vi "BasicExampleMux.vi"() -> ()   [LabVIEW 2025]
uses:
  PalmSens/PalmSens.lvclass
  C:/Users/stef/code/palmsenssdk/labview/PalmSens/Libraries/PalmSens.Core.Simplified.LabVIEW.dll
  PalmSens/Libraries/PalmSens.Core.Simplified.LabVIEW.dll
  PalmSens/MeasurementResults.ctl
  PalmSens/LiveCurveResult.ctl
panel:
  out "NumMuxChannels":i32
  out "Results":T1
  out "LSV Method Indicator":refnum<k24>
  out "Array":string[](array[string])
  out "Is Measuring":bool
  in  "PalmSens.lvclass":refnum<class "PalmSens.lvclass">
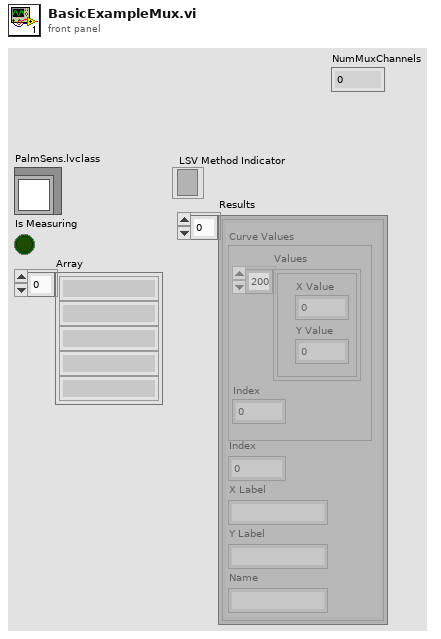
[diagram p1: front panel]
types:
  T1 = typedef "MeasurementResults.ctl" = T2[]
  T2 = typedef "LiveCurveResult.ctl" = cluster{"X Label":string, "Y Label":string, "Name":string, "Index":i16, "Curve Values":cluster{"Values":cluster{"X Value":dbl, "Y Value":dbl}[], "Index":i16}}
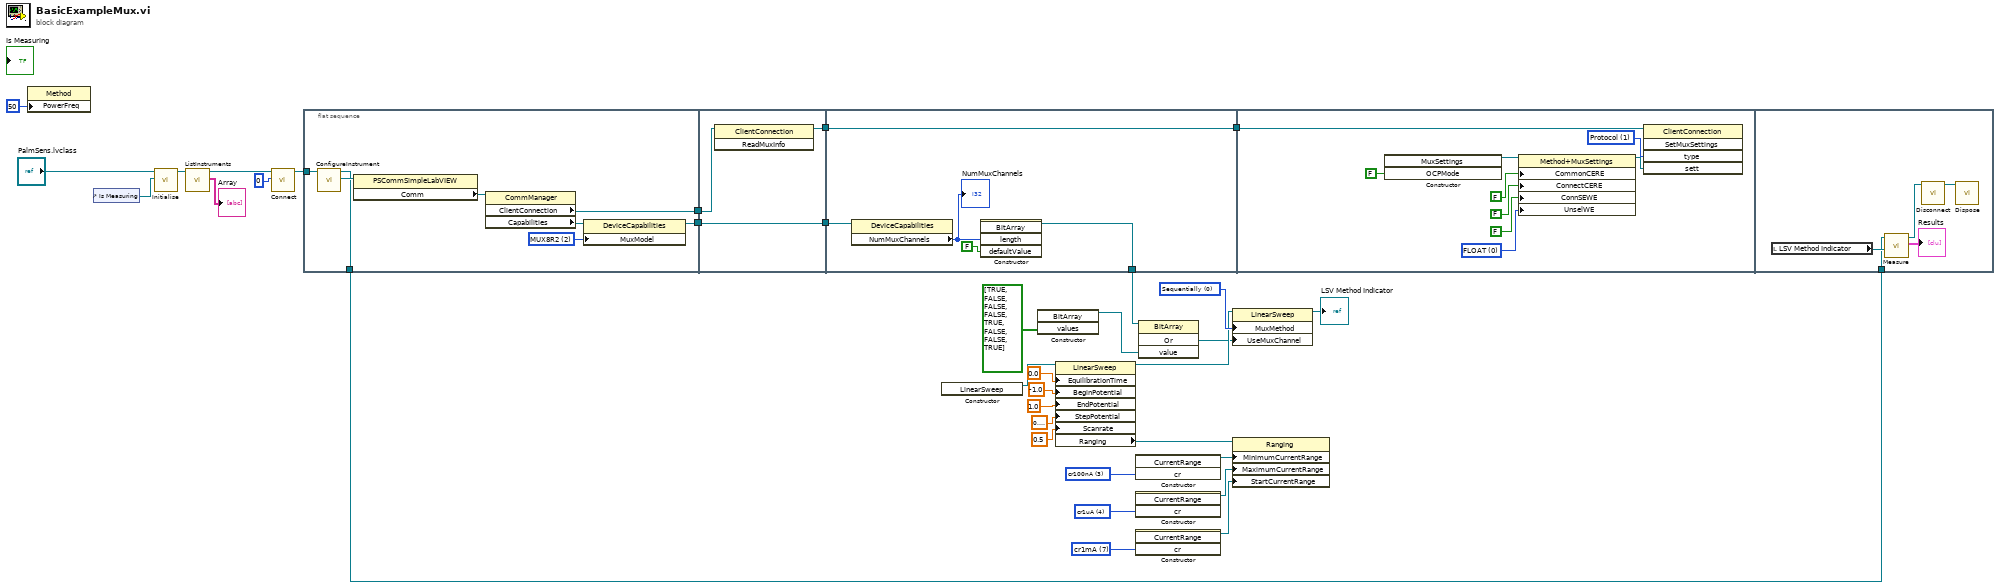
[diagram p0: block diagram]
diagram:
  w22 = 0 items=["Sequentially"=0, "Alternatingly"=1, "None"=-1] ("MuxMethod")
  w25 = 4 items=["cr100pA"=0, "cr1nA"=1, "cr10nA"=2, "cr100nA"=3, "cr1uA"=4, "cr10uA"=5, "cr100uA"=6, "cr1mA"=7, "cr10mA"=8, "cr100mA"=9, "cr2uA"=10, "cr4uA"=11, "cr8uA"=12, "cr16uA"=13, "cr32uA"=14, "cr125uA"=17, "cr250uA"=18, "cr500uA"=19, "cr5mA"=20, "cr6uA"=21, "cr13uA"=22, "cr25uA"=23, "cr50uA"=24, "cr200uA"=25, "cr63uA"=26] ("cr")
  w26 = 7 items=["cr100pA"=0, "cr1nA"=1, "cr10nA"=2, "cr100nA"=3, "cr1uA"=4, "cr10uA"=5, "cr100uA"=6, "cr1mA"=7, "cr10mA"=8, "cr100mA"=9, "cr2uA"=10, "cr4uA"=11, "cr8uA"=12, "cr16uA"=13, "cr32uA"=14, "cr125uA"=17, "cr250uA"=18, "cr500uA"=19, "cr5mA"=20, "cr6uA"=21, "cr13uA"=22, "cr25uA"=23, "cr50uA"=24, "cr200uA"=25, "cr63uA"=26] ("cr")
  w28 = 3 items=["cr100pA"=0, "cr1nA"=1, "cr10nA"=2, "cr100nA"=3, "cr1uA"=4, "cr10uA"=5, "cr100uA"=6, "cr1mA"=7, "cr10mA"=8, "cr100mA"=9, "cr2uA"=10, "cr4uA"=11, "cr8uA"=12, "cr16uA"=13, "cr32uA"=14, "cr125uA"=17, "cr250uA"=18, "cr500uA"=19, "cr5mA"=20, "cr6uA"=21, "cr13uA"=22, "cr25uA"=23, "cr50uA"=24, "cr200uA"=25, "cr63uA"=26] ("cr")
  n1 = property class="Method"("PowerFreq"=50) -> ()  [unwired: 2 in, 2 out]
  n2 = control-ref of="Is Measuring"() -> (w33:refnum<vi>)
  n3 = call-dynamic "Initialise.vi"("Is Measuring Refnum"=w33, "PalmSens in"="PalmSens.lvclass") -> ("PalmSens out"=w32:refnum<class "PalmSens.lvclass">)  [unwired: 8 in, 1 out]
  n4 = call-dynamic "ListInstruments.vi"("PalmSens in"=w32) -> ("Array"=→"Array":string[], "PalmSens out"=w30:refnum<class "PalmSens.lvclass">)  [unwired: 8 in, 1 out]
  n5 = call-dynamic "Connect.vi"("Instrument Index"=0, "PalmSens in"=w30) -> ("PalmSens out"=w2:refnum<class "PalmSens.lvclass">)  [unwired: 8 in, 1 out]
  n6 = flat-sequence {
    tunnel: [w39] -> w11
    tunnel: [w38] -> w8
    tunnel: w2 -> [w37]
    tunnel: [w35] -> w1
    tunnel: [w44] -> w10
    tunnel: w11 -> [w45]
    tunnel: w8 -> [w43]
    tunnel: [w43] -> w7
    tunnel: w10 -> [w50]
    tunnel: [w50] -> w9
    tunnel: w7 -> [w49]
    tunnel: [w46] -> w5
    tunnel: w9 -> [w51]
    tunnel: w1 -> [w60]
    frame #0 {
      w40 = 2 items=["MUX8", "MUX16", "MUX8R2", "PicoMUX16", "PicoMUX256"] ("MuxModel")
      n7 = call-dynamic "ConfigureInstrument.vi"("PalmSens in"=w37) -> ("PSLabView Instance"=w36:refnum<k24>, "PalmSens out"=w35:refnum<class "PalmSens.lvclass">)  [unwired: 8 in, 1 out]
      n8 = property class="PSCommSimpleLabVIEW"(reference=w36) -> ("Comm"=w41:refnum<k24>)  [unwired: 1 in, 2 out]
      n9 = property class="CommManager"(reference=w41) -> ("ClientConnection"=w39:refnum<k24>, "Capabilities"=w42:refnum<k24>)  [unwired: 1 in, 2 out]
      n10 = property class="DeviceCapabilities"(reference=w42, "MuxModel"=w40) -> (reference out=w38:refnum<k24>)  [unwired: 1 in, 1 out]
    }
    frame #1 {
      n11 = invoke class="ClientConnection" method="ReadMuxInfo"(reference=w45) -> (reference out=w44:refnum<k24>)  [unwired: 2 in, 2 out]
    }
    frame #2 {
      n12 = property class="DeviceCapabilities"(reference=w49) -> ("NumMuxChannels"=w48:i32)  [unwired: 1 in, 2 out]
      "NumMuxChannels" <- w48
      n13 = constructor class="BitArray"("length"=w48, "defaultValue"=FALSE) -> (reference out=w46:refnum<k24>)  [unwired: 3 in, 4 out]
    }
    frame #3 {
      w54 = 0 items=["FLOAT", "GND", "VSTDBY"] ("UnselWE")
      w52 = 1 items=["AuxAddress", "Protocol"] ("type")
      n14 = constructor class="Method+MuxSettings"("OCPMode"=FALSE) -> (reference out=w58:refnum<k24>)  [unwired: 3 in, 3 out]
      n15 = property class="Method+MuxSettings"(reference=w58, "CommonCERE"=FALSE, "ConnectCERE"=FALSE, "ConnSEWE"=FALSE, "UnselWE"=w54) -> (reference out=w59:refnum<k24>)  [unwired: 1 in, 1 out]
      n16 = invoke class="ClientConnection" method="SetMuxSettings"(reference=w51, "type"=w52, "sett"=w59) -> ()  [unwired: 2 in, 5 out]
    }
    frame #4 {
      n17 = local read "LSV Method Indicator"() -> (w64:refnum<k24>)
      n18 = call-dynamic "Measure.vi"("Method .NET Refnum"=w64, "PalmSens in"=w60) -> ("Curves"=→"Results":T1, "PalmSens out"=w63:refnum<class "PalmSens.lvclass">)  [unwired: 2 in, 2 out]
      n19 = call-dynamic "Disconnect.vi"("PalmSens in"=w63) -> ("PalmSens out"=w61:refnum<class "PalmSens.lvclass">)  [unwired: 9 in, 1 out]
      n20 = call-dynamic "Dispose.vi"("PalmSens in"=w61) -> ()  [unwired: 9 in, 2 out]
    }
  }
  n21 = constructor class="LinearSweep"() -> (reference out=w14:refnum<k24>)  [unwired: 3 in, 2 out]
  n22 = constructor class="BitArray"("values"=bool[] [TRUE, FALSE, FALSE, FALSE, TRUE, FALSE, FALSE, TRUE]) -> (reference out=w4:refnum<k24>)  [unwired: 3 in, 3 out]
  n23 = property class="LinearSweep"(reference=w14, "EquilibrationTime"=sgl 0.0, "BeginPotential"=sgl -1.0, "EndPotential"=sgl 1.0, "StepPotential"=sgl 0.1, "Scanrate"=sgl 0.5) -> (reference out=w13:refnum<k24>, "Ranging"=w15:refnum<k24>)  [unwired: 1 in, 1 out]
  n24 = constructor class="CurrentRange"("cr"=w28) -> (reference out=w27:refnum<k24>)  [unwired: 3 in, 3 out]
  n25 = constructor class="CurrentRange"("cr"=w25) -> (reference out=w21:refnum<k24>)  [unwired: 3 in, 3 out]
  n26 = constructor class="CurrentRange"("cr"=w26) -> (reference out=w20:refnum<k24>)  [unwired: 3 in, 3 out]
  n27 = invoke class="BitArray" method="Or"(reference=w5, "value"=w4) -> ("Or"=w3:refnum<k24>)  [unwired: 2 in, 3 out]
  n28 = property on="Property Node" class="LinearSweep"(reference=w13, "MuxMethod"=w22, "UseMuxChannel"=w3) -> (reference out=→"LSV Method Indicator":refnum<k24>)  [unwired: 1 in, 1 out]
  n29 = property class="Ranging"(reference=w15, "MinimumCurrentRange"=w27, "MaximumCurrentRange"=w21, "StartCurrentRange"=w20) -> ()  [unwired: 1 in, 2 out]
